vi "Export To File.vi"(8 "error in (no error)":errorcluster, 11 "Node Ptr":u64 format="%.0x") -> (0 "error out":errorcluster)   [LabVIEW 2013, in "MUX Custom Device.lvlib"]
uses:
  MUX Custom Device.lvlib
panel:
  in  "MUX Configuration Path":path
  in  "Cancel":bool
  in  "OK":bool
  in  "Tag":string
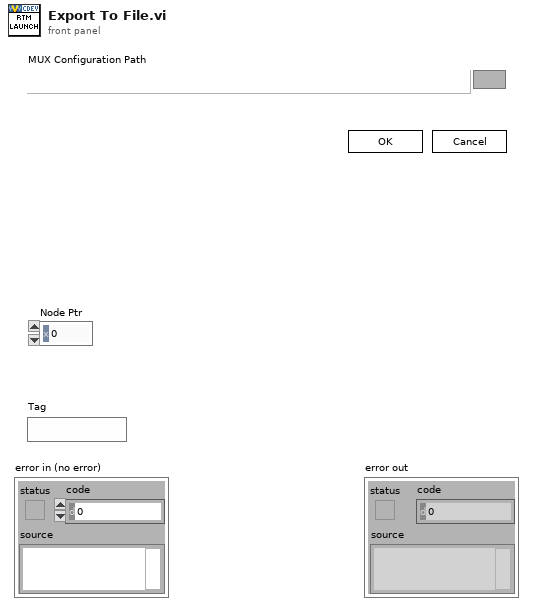
[diagram p1: front panel]
types:
  T1 = enum8{"Enabled", "Disabled", "Disabled and Grayed Out"}
  T2 = typedef "MUX Custom Device.lvlib/Mux Data.ctl" = cluster{"Mux Name":string, "Relay Channel Data":T3[]}
  T3 = typedef "MUX Custom Device.lvlib/Relay Channel Data.ctl" = cluster{"Relay Channel Name":string, "Relay Data":T4}
  T4 = typedef "MUX Custom Device.lvlib/Relay Data.ctl" = cluster{"Relay Name":string, "State":T5}
  T5 = typedef "MUX Custom Device.lvlib/Switch.ctl" = bool
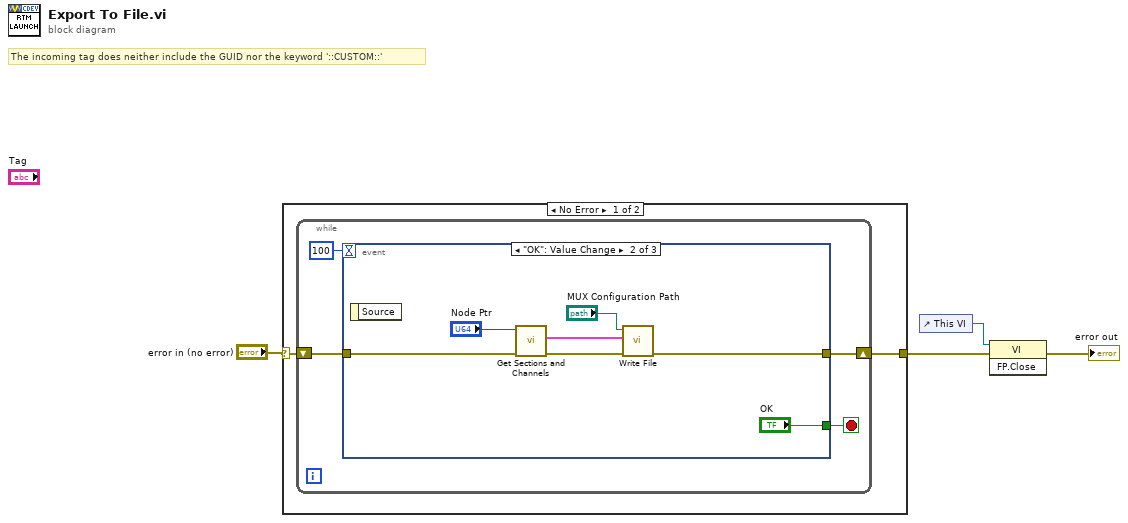
[diagram p0: block diagram]
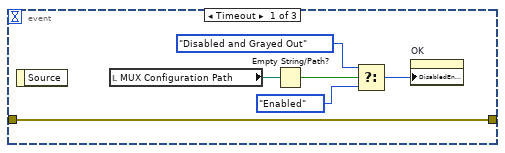
[diagram p2: hidden frame]
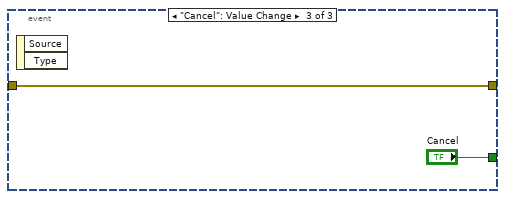
[diagram p3: hidden frame]
diagram:
  # "The incoming tag does neither include the GUID nor the keyword '::CUSTOM::'"
  n1 = case shown="No Error" "error in (no error)" {
    selector: "error in (no error)" -> [w6 w26]
    tunnel: [w5 w26] -> w3
    frame No Error {
      n2 = while {
        shift-right: [w8] -> w5
        shift-left: w6 -> [w9]
        stop <- w7 stop-if-true
        n3 = event shown="[1] \"OK\": Value Change" {
          selector: _ -> [_ _ _]
          dyn-events: _ -> [_ _ _]
          timeout: 100 -> [_ _ _]
          tunnel: w9 -> [w11 w23 w25]
          tunnel: [w11 w19 w25] -> w8
          tunnel: [_ "OK" "Cancel"] -> w7
          event Timeout {
            n4 = event-data() -> ()  [unwired: 1 in, 1 out]
            n5 = local read "MUX Configuration Path"() -> (w16:path)
            n6 = Empty String/Path?(string/path=w16) -> (empty?=w15:bool)
            n7 = Select(t=T1."Disabled and Grayed Out" ("Disabled"), s=w15, f=T1."Enabled" ("Disabled")) -> (s? t:f=w12:T1)
            n8 = property on="OK" class="Bool"("DisabledEnum"=w12) -> ()  [unwired: 2 in, 2 out]
          }
          event "OK": Value Change {
            n9 = event-data() -> ()  [unwired: 1 in, 1 out]
            n10 = call "Get Sections and Channels.vi"("Error In"=w23, "Custom Device Ref in"="Node Ptr") -> ("Error Out"=w21:errorcluster, "Mux Data Array"=w17:T2[])  [unwired: 7 in, 1 out]
            n11 = call "Write File.vi"("Error In"=w21, "Mux Data Array"=w17, "Mux File Path"="MUX Configuration Path") -> ("Error Out"=w19:errorcluster)  [unwired: 8 in]
          }
          event "Cancel": Value Change {
            n12 = event-data() -> ()  [unwired: 1 in, 2 out]
          }
        }
      }
    }
    frame Error {
    }
  }
  n13 = control-ref of="This VI"() -> (w2:refnum<vi>)
  n14 = invoke class="VI" method="FP.Close"(reference=w2, error in=w3) -> (error out=→"error out":errorcluster)  [unwired: 1 in, 2 out]
